vi "RedistributePathPointsVariable.vi"(1 "DesiredPointSpacing":dbl[](array[numeric]), 2 "PathIn":T1[](array[typedef]), 3 "IndexedPathLength":dbl[](array[numeric])) -> (0 "PathOut":T1[](array[typedef]))   [LabVIEW 2017]
uses:
  TypeDefs/Point2D.ctl
  ArgosLib/ArgosLib.lvlib
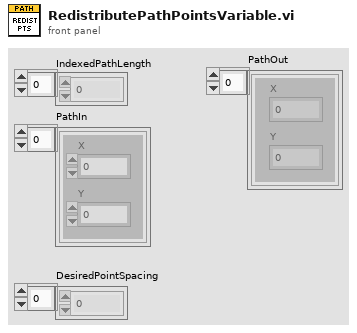
[diagram p1: front panel]
types:
  T1 = typedef "Point2D.ctl" = cluster{"X":dbl, "Y":dbl}
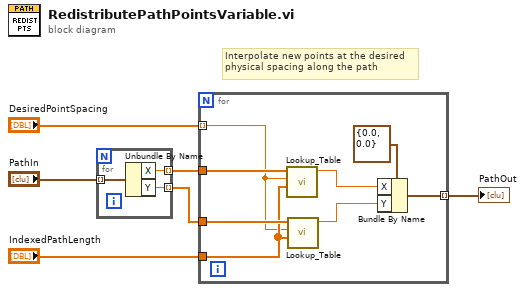
[diagram p0: block diagram]
diagram:
  # "Interpolate new points at the desired\nphysical spacing along the path"
  n1 = for {
    tunnel: "PathIn" -> [w9] mode=indexing
    tunnel: [w8] -> w4 mode=indexing
    tunnel: [w7] -> w3 mode=indexing
    n2 = Unbundle By Name(w9) -> ("X"=w8:dbl, "Y"=w7:dbl)
  }
  n3 = for {
    tunnel: w4 -> [w17]
    tunnel: w3 -> [w16]
    tunnel: "IndexedPathLength" -> [w15]
    tunnel: [w11] -> w2 mode=indexing
    tunnel: "DesiredPointSpacing" -> [w10] mode=indexing
    n4 = call "Lookup_Table.vi"("Y_Array"=w17, "x_in"=w10, "X_Array"=w15) -> ("y_out"=w13:dbl)  [unwired: 6 in]
    n5 = call "Lookup_Table.vi"("Y_Array"=w16, "x_in"=w10, "X_Array"=w15) -> ("y_out"=w12:dbl)  [unwired: 6 in]
    n6 = Bundle By Name(cluster=T1 {"X"=0.0, "Y"=0.0} ("2DPoint"), "X"=w13, "Y"=w12) -> (w11:T1)
  }
  "PathOut" <- w2
